vi "Init.vi"(8 "error in (no error)":errorcluster, 9 "Intrs Configs":T1, 10 "Excitation":T2, 11 "Lock-In Remote Actor in":refnum<class "Lock-In Remote Actor.lvclass">) -> (0 "error out":errorcluster, 3 "Lock-In Remote Actor out":refnum<class "Lock-In Remote Actor.lvclass">)   [LabVIEW 2023, in "Lock-In Remote Actor.lvlib" / "Lock-In Remote Actor.lvclass"]
uses:
  Lock-In Remote Actor.lvclass
  Lock-In Remote Actor.lvclass/Lock-In Remote Actor.ctl
  Interfaces/IMSS Remote Actor/IMSS Remote Actor/IMSS Remote Actor Messages/Init Msg/Init Msg.lvclass/Init Msg.ctl
  <vilib>/ActorFramework/Message Enqueuer/Message Enqueuer.lvclass/Message Enqueuer.ctl
  <vilib>/ActorFramework/Message Enqueuer/Enqueue.vi
  Interfaces/IMSS Remote Actor/IMSS Remote Actor/IMSS Remote Actor Messages/Init Msg/Init Msg.lvclass
  C:/Program Files/National Instruments/LabVIEW 2023/vi.lib/ActorFramework/Message/Message.lvclass
  <vilib>/ActorFramework/Message Priority Queue/Priority Enqueue.vi
  <vilib>/Utility/error.llb/Error Cluster From Error Code.vi
  <vilib>/ErrorRing/Error Ring.xnode
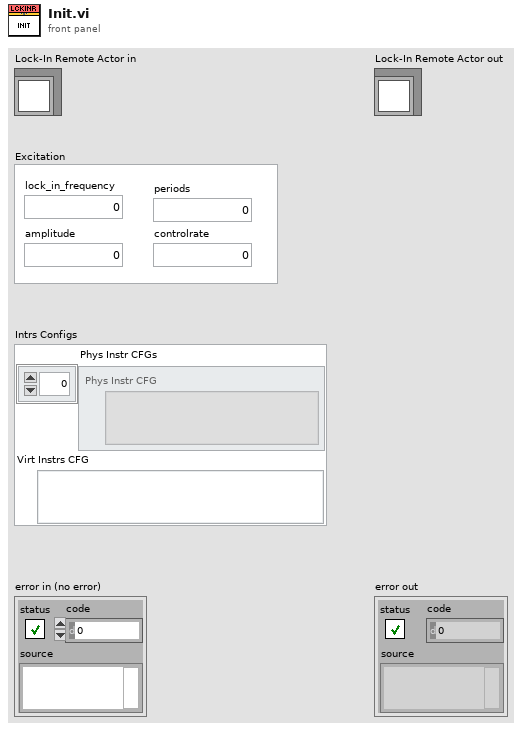
[diagram p1: front panel]
types:
  T1 = cluster{"Phys Instr CFGs":path[], "Virt Instrs CFG":path}
  T2 = cluster{"lock_in_frequency":dbl, "amplitude":dbl, "periods":dbl, "controlrate":dbl}
  T3 = map{string, refnum<class "Message Enqueuer.lvclass">}
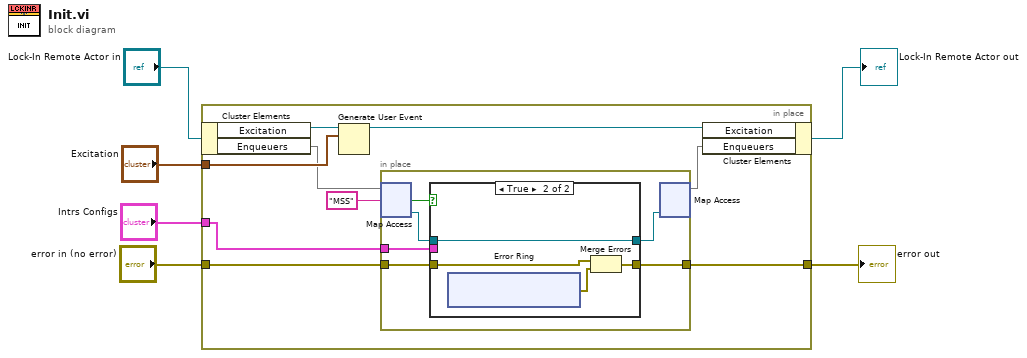
[diagram p0: block diagram]
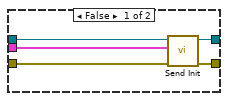
[diagram p2: hidden frame]
diagram:
  n1 = in-place {
    in-place-border: "Excitation" -> [w13]
    in-place-border: "error in (no error)" -> [w10]
    in-place-border: "Intrs Configs" -> [w9]
    in-place-border: [w8] -> w1
    n2 = in-place-cluster #1("Lock-In Remote Actor in") -> ("Excitation"=w15:refnum<user-event>, "Enqueuers"=w12:T3)
    n3 = Generate User Event(user event=w15, event data cluster=w13) -> (user event out=w14:refnum<user-event>)  [unwired: 2 in, 1 out]
    n4 = in-place {
      in-place-border: w10 -> [w21]
      in-place-border: w9 -> [w20]
      in-place-border: [w17] -> w8
      n5 = in-place-map #2(w12, "MSS") -> (w19:refnum<class "Message Enqueuer.lvclass">, w16:bool)  [unwired: 1 in]
      n6 = case shown="True" w16 {
        tunnel: w21 -> [w26 w29]
        tunnel: w20 -> [w25 _]
        tunnel: w19 -> [w24 w27]
        tunnel: [w23 w27] -> w18
        tunnel: [w22 w30] -> w17
        frame False {
          n7 = call "Send Init.vi"("error in (no error)"=w26, "Intrs Configs"=w25, "Message Enqueuer"=w24) -> ("error out"=w22:errorcluster, "Message Enqueuer out"=w23:refnum<class "Message Enqueuer.lvclass">)  [unwired: 7 in]
        }
        frame True {
          n8 = xnode "Error Ring"() -> ("error out"=w28:errorcluster)
          n9 = Merge Errors(w29, w28) -> (w30:errorcluster)
        }
      }
      n10 = in-place-map #2(w18) -> (w7:T3)  [unwired: 1 in, 2 out]
    }
    n11 = in-place-cluster #1("Excitation"=w14, "Enqueuers"=w7) -> (→"Lock-In Remote Actor out":refnum<class "Lock-In Remote Actor.lvclass">)
  }
  "error out" <- w1
